vi "Create JS File.vi"(8 "error in (no error)":errorcluster, 11 "Material Theme in":refnum<class "Material Theme.lvclass">) -> (0 "error out":errorcluster, 3 "Material Theme out":refnum<class "Material Theme.lvclass">)   [LabVIEW 2021, in "TSC Material Theme.lvlib" / "Material Theme.lvclass"]
doc: "I have no recollection of why I made this or what it's purpose is. I am just going to leave it in case it is important........\n\n<b>Code Developed By:</b>\nTechnology Service Corporation\nwww.tsc.com/atcs\n\nDeveloper:\nDaniel Coons"
uses:
  Material Theme.lvclass
  Material Theme.lvclass/Material Theme.ctl
  Material-Scheme/Material-Scheme.lvclass/Material-Scheme.ctl
  Material-Scheme/data member access/Read name.vi
  Material-Scheme/data member access/Read CSS Variables.vi
  Material-Scheme/Material-Scheme.lvclass
panel:
  out "delimited string":string
  out "Array":string[](array[string])
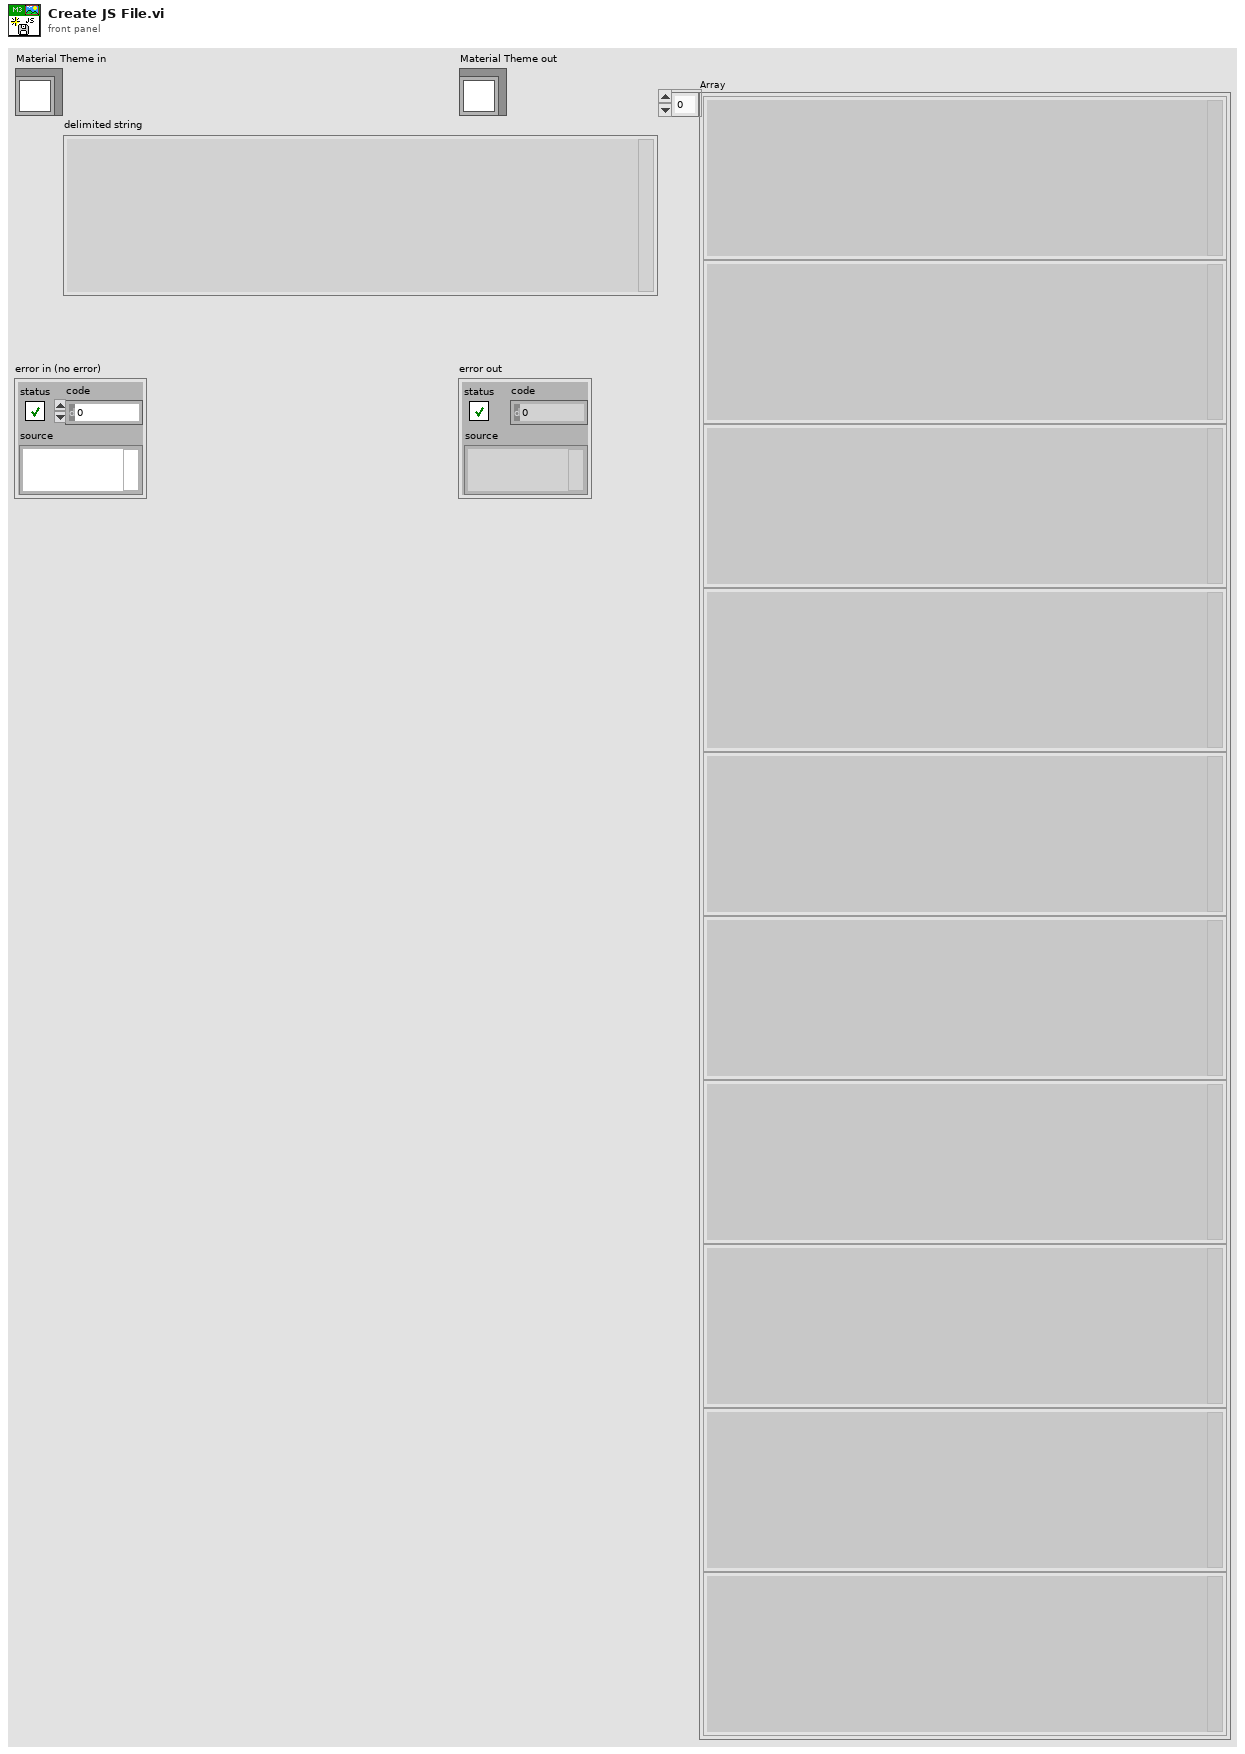
[diagram p1: front panel]
types:
  T1 = enum16{"open", "replace", "create", "open or create", "replace or create", "replace or create with confirmation"}
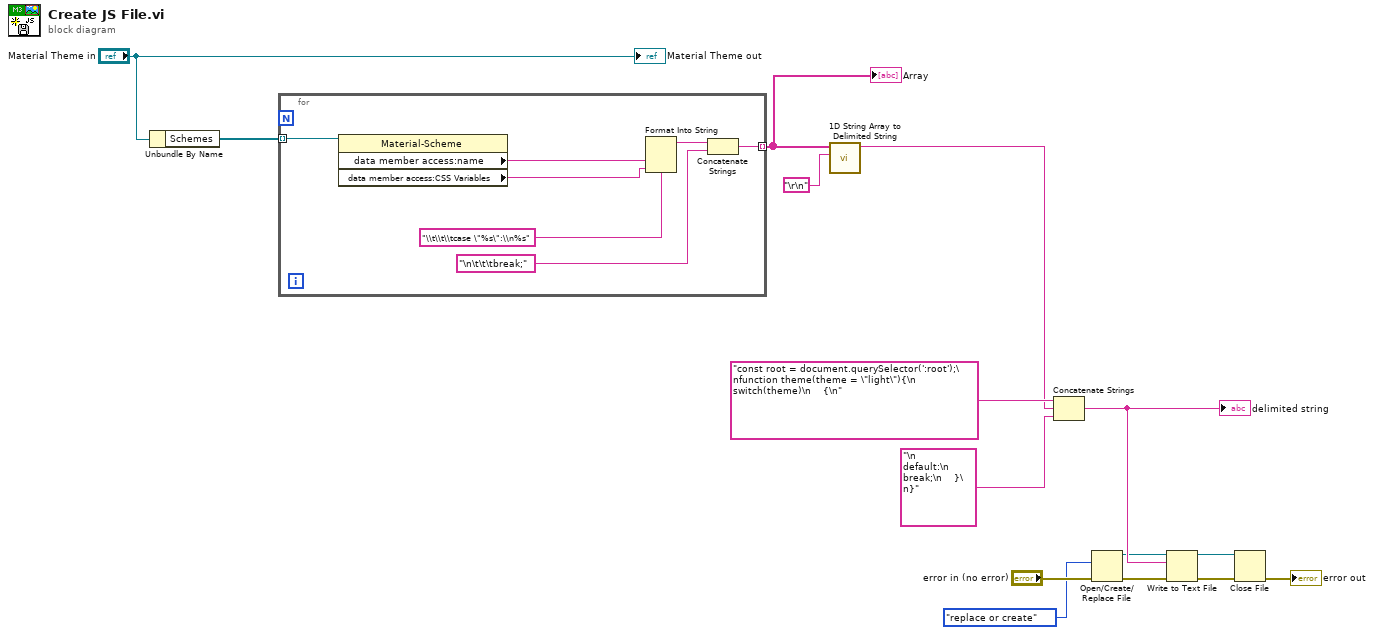
[diagram p0: block diagram]
diagram:
  n1 = Unbundle By Name("Material Theme in") -> ("Schemes"=w10:refnum<class "Material-Scheme.lvclass">[])
  n2 = for {
    tunnel: w10 -> [w22] mode=indexing
    tunnel: [w16] -> w8 mode=indexing
    n3 = property class="Material-Scheme"(reference=w22) -> ("data member access:name"=w20:string, "data member access:CSS Variables"=w19:string)  [unwired: 1 in, 2 out]
    n4 = Format Into String(format string="\\t\\t\\tcase \"%s\":\\n%s", w20, w19) -> (resulting string=w18:string)  [unwired: 2 in, 1 out]
    n5 = Concatenate Strings(w18, "\n\t\t\tbreak;" ("string")) -> (w16:string)
  }
  "Array" <- w8
  n6 = call <vilib>:"1D String Array to Delimited String.vi"("delimiter"="\r\n", "string array"=w8) -> ("delimited string"=w7:string)  [unwired: 9 in]
  n7 = Concatenate Strings("const root = document.querySelector(':root');\nfunction theme(theme = \"light\"){\n    switch(theme)\n    {\n", w7, "\n        default:\n            break;\n    }\n}") -> (w5:string)
  "delimited string" <- w5
  n8 = Open/Create/Replace File(error in="error in (no error)", operation (0:open)=T1."replace or create") -> (refnum out=w2:refnum<file>, error out=w4:errorcluster)  [unwired: 4 in, 1 out]
  n9 = Write to Text File(file (use dialog)=w2, text=w5, error in=w4) -> (refnum out=w1:refnum<file>, error out=w3:errorcluster)  [unwired: 1 in, 1 out]
  n10 = Close File(refnum=w1, error in=w3) -> (error out=→"error out":errorcluster)  [unwired: 1 out]
  "Material Theme out" <- "Material Theme in"
